vi "Index_Meas_Data_Arrays.vi"(4 "2nd Desired Index":i32, 5 "1st Desired Index":i32, 6 "Equi Spaced":dbl[][](array[numeric]) format="%.2f", 7 "Vari Spaced":dbl[][](array[numeric]) format="%.2f") -> (0 "2nd Output Index":i32, 1 "1st Output Index":i32, 2 "Index Offset":i32, 3 "Output Array":dbl[][](array[numeric]) format="%.2f")   [LabVIEW 2010]
uses:
  Controls/Instrument_Array.ctl
  Globals/Meas_global.vi
  Acquisition/PWA/PWAtasksGLOBAL.vi
panel:
  out "Inst Array":T1
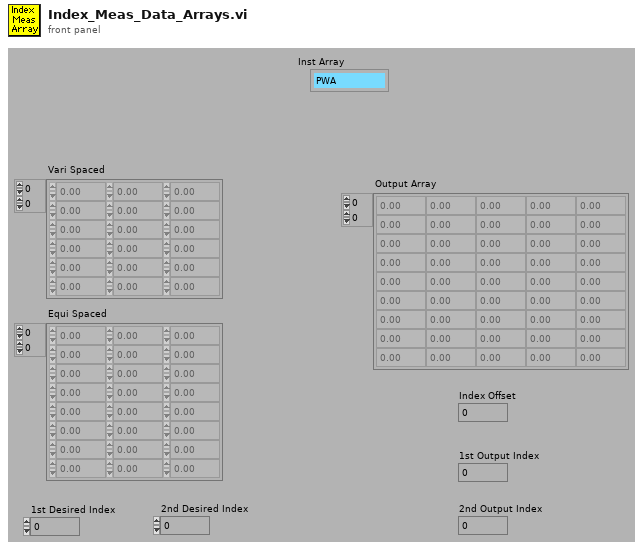
[diagram p1: front panel]
types:
  T1 = typedef "Instrument_Array.ctl" = enum16{"PWA", "LDA", "Analogue"}
  T2 = typedef "Analysis_info_cluster.ctl" = cluster{"Colour":u32, "Inst type":T3, "Inst name":string, "Symbol":string, "Code name":string, "Extra Info":string, "Inst Array":T1, "Index":i32, "Voltage Index":i32, "Extra Titles":string[], "Extra Values":string[]}
  T3 = typedef "Inst_type.ctl" = enum16{"Propeller anemometer", "Raw voltage", "Pressure Transducer", "Pitot-static tube", "Preston tube", "Hot wire", "Cross wire 1", "Cross wire 2", "Generic Linear", "Generic Polynomial", "Generic BackPoly", "Fast FID", "Thermocouple", "Cold wire", "Pulsed Wire", "LDA Vel", "LDA Tran time", "LDA Arr time"}
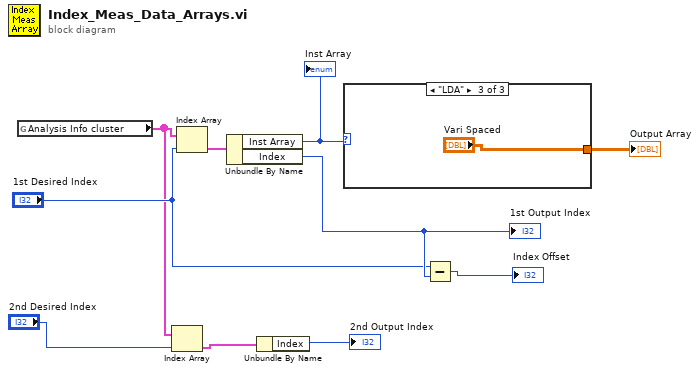
[diagram p0: block diagram]
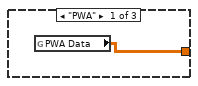
[diagram p2: hidden frame]
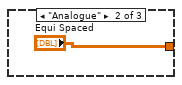
[diagram p3: hidden frame]
diagram:
  n1 = global read "Meas_global.vi" "Analysis Info cluster"() -> (w4:T2[])
  n2 = Index Array(array=w4, index="2nd Desired Index") -> (element=w2:T2)
  n3 = Index Array(array=w4, index="1st Desired Index") -> (element=w10:T2)
  n4 = Unbundle By Name(w10) -> ("Inst Array"=w9:T1, "Index"=w7:i32)
  "1st Output Index" <- w7
  "Inst Array" <- w9
  n5 = Unbundle By Name(w2) -> ("Index"=→"2nd Output Index":i32)
  n6 = case shown="\"LDA\"" w9 {
    tunnel: [w11 "Equi Spaced" "Vari Spaced"] -> w8
    frame "PWA" {
      n7 = global read "PWAtasksGLOBAL.vi" "PWA Data"() -> (w11:dbl[][])
    }
    frame "Analogue" {
    }
    frame "LDA" {
    }
  }
  "Output Array" <- w8
  n8 = Subtract(x="1st Desired Index", y=w7) -> (x-y=→"Index Offset":i32)
